vi "BMark_Get Bookmarks.vi"(8 "error in (no error)":errorcluster, 10 "Reset BM Cache?":bool, 11 "App Info":T1) -> (0 "error out":errorcluster, 1 "All desc":string[](array[string]), 2 "possible undisplayed bookmarks":bool, 3 "bookmarks":T2[](array[typedef]))   [LabVIEW 2018]
uses:
  controls/BMark_Bookmark Data.ctl
  controls/BMark_VI_Identifier.ctl
  <vilib>/addons/analyzer/_analyzerctrls.llb/VIAnCtl Analysis App Info.ctl
panel:
  out "Class Desc":string[](array[string])
  out "Lib desc":string[](array[string])
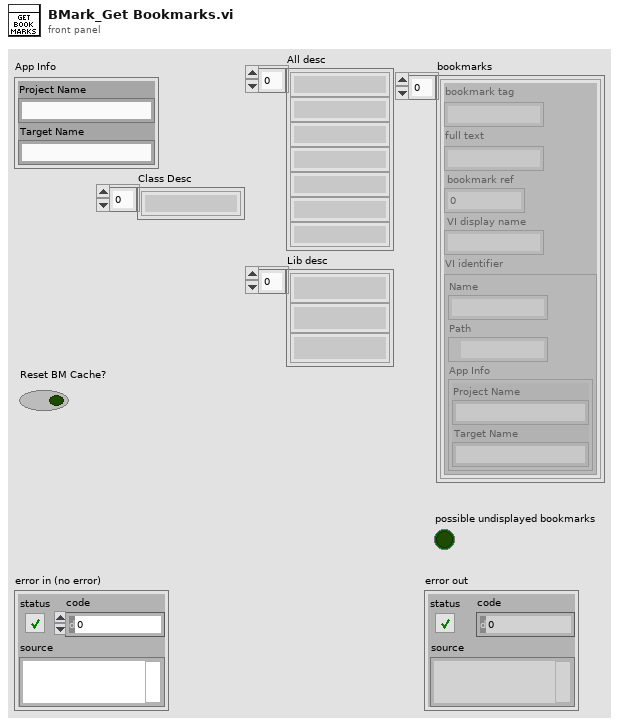
[diagram p1: front panel]
types:
  T1 = typedef "VIAnCtl Analysis App Info.ctl" = cluster{"Project Name":string, "Target Name":string}
  T2 = typedef "BMark_Bookmark Data.ctl" = cluster{"bookmark tag":string, "full text":string, "bookmark ref":i32, "VI display name":string, "VI identifier":T3}
  T3 = typedef "BMark_VI_Identifier.ctl" = cluster{"Name":string, "Path":path, "App Info":T1}
  T4 = typedef "LVBookmarkInfoTypeDef.ctl" = cluster{"Bookmark ID":u32, "Bookmark Tag":string, "Label Text":string}[]
  T5 = typedef "BMark_Array of Bookmarks.ctl" = T6[]
  T6 = typedef "BMark_Bookmark Cluster.ctl" = cluster{"bookmark ref":i32, "bookmark":string, "label text":string, "VI identifier":T3}
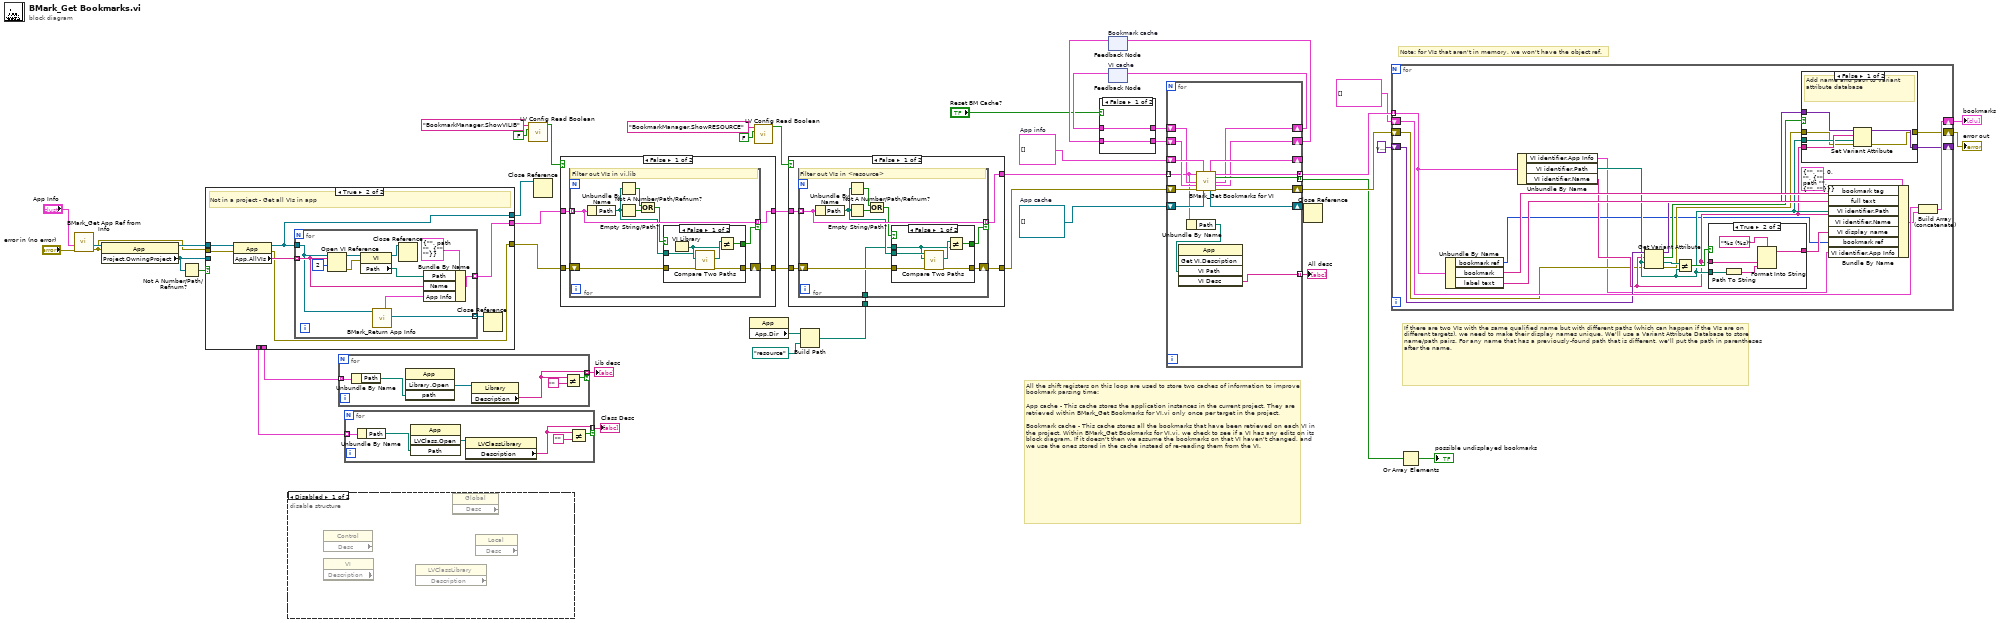
[diagram p0: block diagram]
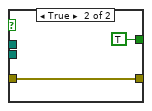
[diagram p4: hidden frame]
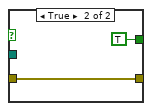
[diagram p6: hidden frame]
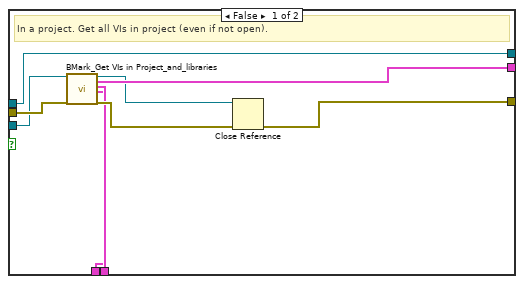
[diagram p8: hidden frame]
diagram:
  w14 = refnum<vi>[] []  # App cache
  w15 = T1[] []  # App info
  # "All the shift registers on this loop are used to store two caches of information to improve bookmark parsing time:\n\nApp cache - This cache stores the application instances in the current project. They are retrieved within BMark_Get Bookmarks for VI.vi only once per target in the project.\n\nBookmark cache - This cache stores all the bookmarks that have been retrieved on each VI in the project. Within BMark_Get Bookmarks for VI.vi, we check to see if a VI has any edits on its block diagram. If it doesn't then we assume the bookmarks on that VI haven't changed, and we use the ones stored in the cache instead of re-reading them from the VI."
  # "Note: for VIs that aren't in memory, we won't have the object ref."
  # "If there are two VIs with the same qualified name but with different paths (which can happen if the VIs are on different targets), we need to make their display names unique. We'll use a Variant Attribute Database to store name/path pairs. For any name that has a previously-found path that is different, we'll put the path in parentheses after the name."
  n1 = call "BMark_Get App Ref from Info.vi"("error in (no error)"="error in (no error)", "Analysis App Info"="App Info") -> ("error out"=w30:errorcluster, "Analysis App ref"=w32:refnum<vi>)  [unwired: 8 in]
  n2 = property class="App"(reference=w32, error in=w30) -> (reference out=w44:refnum<vi>, "Project.OwningProject"=w43:refnum<vi>)  [unwired: 1 out]
  n3 = Not A Number/Path/Refnum?(number/path/refnum=w43) -> (NaN/Path/Refnum?=w45:bool)
  n4 = case shown="True" w45 {
    tunnel: w44 -> [w53 w62]
    tunnel: w43 -> [w51 _]
    tunnel: [w49 w58] -> w23
    tunnel: w30 -> [w55 w61]
    tunnel: [w54 w59] -> w22
    tunnel: [w53 w57] -> w29
    tunnel: [w48 _] -> w5
    tunnel: [w47 _] -> w2
    frame False {
      # "In a project. Get all VIs in project (even if not open)."
      n5 = call "BMark_Get VIs in Project_and_libraries.vi"("project"=w51, "error in (no error)"=w55) -> ("project out"=w50:refnum<vi>, "Array of VIs"=w54:T3[], "Library"=w48:T3[], "LVClassLibrary"=w47:T3[], "error out"=w52:errorcluster)  [unwired: 11 in, 2 out]
      n6 = Close Reference(reference=w50, error in (no error)=w52) -> (error out=w49:errorcluster)
    }
    frame True {
      # "Not in a project - Get all VIs in app"
      n7 = property class="App"(reference=w62, error in=w61) -> (reference out=w57:refnum<vi>, error out=w58:errorcluster, "App.AllVIs"=w60:string[])
      n8 = for {
        tunnel: w60 -> [w68] mode=indexing
        tunnel: [w72] -> w59 mode=indexing
        tunnel: w57 -> [w67]
        tunnel: [w64] -> w56 mode=indexing
        n9 = Open VI Reference(application reference (local)=w67, vi path=w68, options=2) -> (vi reference=w71:refnum<vi>, error out=w70:errorcluster)  [unwired: 3 in]
        n10 = property class="VI"(reference=w71, error in=w70) -> (reference out=w65:refnum<vi>, "Path"=w69:path)  [unwired: 1 out]
        n11 = call "BMark_Return App Info.vi"("App Refnum in"=w67) -> ("App Refnum for Opening VI"=w64:refnum<vi>, "App Info"=w66:T1)  [unwired: 8 in, 1 out]
        n12 = Close Reference(reference=w65) -> ()  [unwired: 1 in, 1 out]
        n13 = Bundle By Name(cluster=T3 {"Name"="", "Path"=path "", "App Info"={"Project Name"="", "Target Name"=""}} ("Cluster"), "Path"=w69, "Name"=w68, "App Info"=w66) -> (w72:T3)
      }
      n14 = Close Reference(reference=w56) -> ()  [unwired: 1 in, 1 out]
    }
  }
  n15 = disable-structure shown="Disabled" {
    frame Disabled {
      n16 = property class="Control" props=["Desc"]() -> ()  [unwired: 2 in, 3 out]
      n17 = property class="VI" props=["Description"]() -> ()  [unwired: 2 in, 3 out]
      n18 = property class="LVClassLibrary" props=["Description"]() -> ()  [unwired: 2 in, 3 out]
      n19 = property class="Global" props=["Desc"]() -> ()  [unwired: 2 in, 3 out]
      n20 = property class="Local" props=["Desc"]() -> ()  [unwired: 2 in, 3 out]
    }
    frame Enabled {
    }
  }
  n21 = for {
    tunnel: w5 -> [w79] mode=indexing
    tunnel: [w74] -> w3 mode=indexing if=w75
    n22 = Unbundle By Name(w79) -> ("Path"=w78:path)
    n23 = invoke class="App" method="Library.Open"("path"=w78) -> ("Open Library"=w77:refnum<vi>)  [unwired: 3 in, 3 out]
    n24 = property class="Library"(reference=w77) -> ("Description"=w74:string)  [unwired: 1 in, 2 out]
    n25 = Not Equal?(x=w74, y="") -> (x != y?=w75:bool)
  }
  "Lib desc" <- w3
  n26 = for {
    tunnel: w2 -> [w85] mode=indexing
    tunnel: [w80] -> w1 mode=indexing if=w81
    n27 = Unbundle By Name(w85) -> ("Path"=w84:path)
    n28 = invoke class="App" method="LVClass.Open"("Path"=w84) -> ("LVClass.Open"=w83:refnum<vi>)  [unwired: 3 in, 3 out]
    n29 = property class="LVClassLibrary"(reference=w83) -> ("Description"=w80:string)  [unwired: 1 in, 2 out]
    n30 = Not Equal?(x=w80, y="") -> (x != y?=w81:bool)
  }
  "Class Desc" <- w1
  n31 = call <resource>:"LV Config Read Boolean.vi"("default value"=FALSE, "key"="BookmarkManager.ShowVILIB") -> ("value"=w37:bool)  [unwired: 3 in, 2 out]
  n32 = Close Reference(reference=w29) -> ()  [unwired: 1 in, 1 out]
  n33 = case shown="False" w37 {
    tunnel: w23 -> [w89 w107]
    tunnel: [w87 w107] -> w27
    tunnel: w22 -> [w88 w106]
    tunnel: [w86 w106] -> w24
    frame False {
      n34 = for {
        shift-right: [w96] -> w87
        shift-left: w89 -> [w97]
        tunnel: w88 -> [w94] mode=indexing
        tunnel: [w94] -> w86 mode=indexing if=w95
        # "Filter out VIs in vi.lib"
        n35 = Unbundle By Name(w94) -> ("Path"=w93:path)
        n36 = Not A Number/Path/Refnum?(number/path/refnum=w93) -> (NaN/Path/Refnum?=w92:bool)
        n37 = Empty String/Path?(string/path=w93) -> (empty?=w91:bool)
        n38 = Or(x=w92, y=w91) -> (x .or. y?=w90:bool)
        n39 = case shown="False" w90 {
          tunnel: w97 -> [w101 w104]
          tunnel: [w100 w104] -> w96
          tunnel: w93 -> [w99 _]
          tunnel: [w98 TRUE] -> w95
          frame False {
            n40 = VI Library() -> (path=w102:path)
            n41 = call <vilib>:"Compare Two Paths.vi"("error in (no error)"=w101, "Path 2"=w102, "Path 1"=w99) -> ("error out"=w100:errorcluster, "Common Path"=w103:path)  [unwired: 5 in, 2 out]
            n42 = Not Equal?(x=w103, y=w102) -> (x != y?=w98:bool)
          }
          frame True {
          }
        }
      }
    }
    frame True {
    }
  }
  n43 = property class="App"() -> ("App.Dir"=w18:path)  [unwired: 2 in, 2 out]
  n44 = call <resource>:"LV Config Read Boolean.vi"("default value"=FALSE, "key"="BookmarkManager.ShowRESOURCE") -> ("value"=w19:bool)  [unwired: 3 in, 2 out]
  n45 = Build Path(base path=w18, name or relative path=path "resource") -> (appended path=w16:path)
  n46 = case shown="False" w19 {
    tunnel: w27 -> [w112 w131]
    tunnel: [w110 w131] -> w26
    tunnel: w24 -> [w111 w130]
    tunnel: [w109 w130] -> w25
    tunnel: w16 -> [w108 _]
    frame False {
      n47 = for {
        shift-right: [w120] -> w110
        shift-left: w112 -> [w121]
        tunnel: w111 -> [w118] mode=indexing
        tunnel: [w118] -> w109 mode=indexing if=w119
        tunnel: w108 -> [w113]
        # "Filter out VIs in <resource>"
        n48 = Unbundle By Name(w118) -> ("Path"=w117:path)
        n49 = Not A Number/Path/Refnum?(number/path/refnum=w117) -> (NaN/Path/Refnum?=w116:bool)
        n50 = Empty String/Path?(string/path=w117) -> (empty?=w115:bool)
        n51 = Or(x=w116, y=w115) -> (x .or. y?=w114:bool)
        n52 = case shown="False" w114 {
          tunnel: w121 -> [w126 w128]
          tunnel: [w125 w128] -> w120
          tunnel: w117 -> [w124 _]
          tunnel: [w123 TRUE] -> w119
          tunnel: w113 -> [w122 _]
          frame False {
            n53 = call <vilib>:"Compare Two Paths.vi"("error in (no error)"=w126, "Path 2"=w122, "Path 1"=w124) -> ("error out"=w125:errorcluster, "Common Path"=w127:path)  [unwired: 5 in, 2 out]
            n54 = Not Equal?(x=w127, y=w122) -> (x != y?=w123:bool)
          }
          frame True {
          }
        }
      }
    }
    frame True {
    }
  }
  n55 = feedback #1 "Bookmark cache"() -> (w8:cluster{"BookmarkInfo":T4}[])  [unwired: 1 in]
  n56 = feedback #2 "VI cache"() -> (w10:T3[])  [unwired: 1 in]
  n57 = case shown="False" "Reset BM Cache?" {
    tunnel: [w133 _] -> w11
    tunnel: w10 -> [w133 _]
    tunnel: [w132 _] -> w9
    tunnel: w8 -> [w132 _]
    frame False {
    }
    frame True {
    }
  }
  n58 = for {
    shift-right: [w147] -> w41
    shift-left: w26 -> [w148]
    tunnel: [w146] -> w42 mode=concatenating
    tunnel: w25 -> [w136] mode=indexing
    tunnel: [w145] -> w35 mode=indexing
    shift-right: [w143] -> _
    shift-left: w15 -> [w144]
    shift-right: [w141] -> w13
    shift-left: w14 -> [w142]
    shift-right: [w140] -> w12
    shift-left: w11 -> [w138]
    shift-right: [w139] -> w6
    shift-left: w9 -> [w137]
    tunnel: [w134] -> w4 mode=indexing
    n59 = Unbundle By Name(w136) -> ("Path"=w135:path)
    n60 = invoke class="App" method="Get VI.Description"("VI Path"=w135) -> ("VI Desc"=w134:string)  [unwired: 4 in, 4 out]
    n61 = call "BMark_Get Bookmarks for VI.vi"("VI"=w136, "App Infos in"=w144, "VI Cache in"=w138, "Bookmark Cache in"=w137, "error in (no error)"=w148, "App cache in"=w142) -> ("App Infos out"=w143:T1[], "Array of bookmarks"=w146:T5, "possible undisplayed bookmarks"=w145:bool, "VI Cache out"=w140:T3[], "Bookmark Cache out"=w139:cluster{"BookmarkInfo":T4}[], "App cache out"=w141:refnum<vi>[], "error out"=w147:errorcluster)  [unwired: 3 in]
  }
  "All desc" <- w4
  n62 = feedback-in #1(w6) -> ()
  n63 = feedback-in #2(w12) -> ()
  n64 = Close Reference(reference=w13) -> ()  [unwired: 1 in, 1 out]
  n65 = for {
    shift-right: [w168] -> w46
    shift-left: T2[] [] -> [w169]
    tunnel: w42 -> [w154] mode=indexing
    shift-right: [w155] -> w40
    shift-left: w41 -> [w151]
    shift-right: [w163] -> _
    shift-left: variant -> [w162]
    n66 = Unbundle By Name(w154) -> ("bookmark ref"=w150:i32, "bookmark"=w164:string, "label text"=w165:string)
    n67 = Unbundle By Name(w154) -> ("VI identifier.App Info"=w149:T1, "VI identifier.Path"=w153:path, "VI identifier.Name"=w152:string)
    n68 = Get Variant Attribute(Variant=w162, name=w152, default value (empty Variant)=w153, error in=w151) -> (duplicate Variant=w158:variant, found=w157:bool, value=w161:path, error out=w156:errorcluster)
    n69 = Not Equal?(x=w161, y=w153) -> (x != y?=w159:bool)
    n70 = case shown="True" w159 {
      tunnel: w153 -> [_ w181]
      tunnel: w152 -> [w178 w180]
      tunnel: [w178 w179] -> w160
      frame False {
      }
      frame True {
        n71 = Path To String(path=w181) -> (string=w182:string)
        n72 = Format Into String(format string="%s (%s)", w180, w182) -> (resulting string=w179:string)  [unwired: 2 in, 1 out]
      }
    }
    n73 = case shown="False" w157 {
      tunnel: [w175 w177] -> w163
      tunnel: w158 -> [w174 w177]
      tunnel: w152 -> [w173 _]
      tunnel: w153 -> [w172 _]
      tunnel: w156 -> [w171 w176]
      tunnel: [w170 w176] -> w155
      frame False {
        # "Add name and path to variant attribute database"
        n74 = Set Variant Attribute(Variant=w174, name=w173, value=w172, error in=w171) -> (Variant out=w175:variant, error out=w170:errorcluster)  [unwired: 1 out]
      }
      frame True {
      }
    }
    n75 = Bundle By Name(cluster=T2 {"bookmark tag"="", "full text"="", "bookmark ref"=0, "VI display name"="", "VI identifier"={"Name"="", "Path"=path "", "App Info"={"Project Name"="", "Target Name"=""}}} ("bookmark item"), "bookmark tag"=w164, "full text"=w165, "VI identifier.Path"=w153, "VI identifier.Name"=w152, "VI display name"=w160, "bookmark ref"=w150, "VI identifier.App Info"=w149) -> (w166:T2)
    n76 = Build Array (concatenate)(w169, w166) -> (w168:T2[])
  }
  "bookmarks" <- w46
  "error out" <- w40
  n77 = Or Array Elements(Boolean array=w35) -> (logical OR=→"possible undisplayed bookmarks":bool)
